vi "EPTxRTmul-inj2.0.vi"(0 "PatternConfig":T14 {"Max Rate [Hz]" format="%#_3p"}, 1 "EPTxFilters":T15={"Primary [s]"=5e-06, "Aux 1 [s]"=5e-06, "Aux 2 [s]"=0.0, "Aux 3 [s]"=0.0, "Aux 4 [s]"=0.0} {"Aux 4 [s]" format="%#_6p"; "Aux 3 [s]" format="%#_6p"; "Aux 2 [s]" format="%#_6p"; "Aux 1 [s]" format="%#_6p"; "Primary [s]" format="%#_6p"}, 5 "RT_Input":T4={"Load"=FALSE, "History_[CAD]"=63, "Stall_Speed_[RPM]"=200.0, "Delay_time[ms]"=0.0} caption="簇", 9 "EPTxState":T17={"Sync Enable"=TRUE, "Clear Errors"=FALSE, "Sim Enable"=FALSE, "Sim Speed [RPM]"=1000.0}, 11 "SimulatorConfig":T13={"Sim Speed [RPM]"=1000.0, "Ramp Rate [RPM/s]"=50.0, "Rotations"=2, "Pause"=FALSE, "Pause Angle [CAD]"=0.0, "Max Offset [RPM]"=0.0, "Cylinders"=6}, 12 "EPTxSupervisor_rt":T9={"Sync"=FALSE, "CurrentCAD"=0.0, "MaxCAD"=720.0, "HistoryCAD"=61.0, "CADRate"=0.0, "AvgSpeed"=0.0, "Config"=FALSE, "Rcvg Primary"=FALSE, "Stall"=FALSE, "Overflow"=FALSE, "Ratio Error"=FALSE, "Pattern Error"=FALSE, "Aux Warning"=FALSE, "Watchdog Error"=FALSE}, 13 "Control_strategy_input":T3={"Injection_DBTDC"=6.0, "Injection_duration[ms]"=2.0} caption="簇") -> (3 "EPTxControl":T10={"Sync Enable"=FALSE, "Clear Errors"=FALSE, "Sim Enable"=FALSE, "Sim Rate"=63.999996185302734, "Watchdog"=FALSE}, 4 "Config_number":T7 caption="簇", 6 "Lighting":T8 caption="簇", 10 "EPTxPatternConfig":T11 {"Pattern"."Aux 4" format="%#_16g"; "Pattern"."Aux 3" format="%#_16g"; "Pattern"."Aux 2" format="%#_16g"; "Pattern"."Aux 1" format="%#_16g"; "Pattern"."Primary" format="%#_16g"}, 14 "CylinderSig":T2={"CylinderSig_1"={"Cylinder1_H_R[CAD]"=204.0, "Cylinder1_H_F[CAD]"=210.0}, "CylinderSig_2"={"Cylinder2_H_R[CAD]"=684.0, "Cylinder2_H_F[CAD]"=690.0}, "CylinderSig_3"={"Cylinder3_H_R[CAD]"=444.0, "Cylinder3_H_F[CAD]"=450.0}, "CylinderSig_4"={"Cylinder4_H_R[CAD]"=90.0, "Cylinder4_H_F[CAD]"=100.0}, "CylinderSig_5"={"Cylinder5_H_R[CAD]"=324.0, "Cylinder5_H_F[CAD]"=330.0}, "CylinderSig_6"={"Cylinder6_H_R[CAD]"=0.0, "Cylinder6_H_F[CAD]"=0.0}} caption="簇", 15 "Tick_output":T1 caption="簇")   [LabVIEW 2022 SP3]
uses:
  <vilib>/Powertrain Controls/Device Drivers/Engine Position Tracking/EPTx/RevA/RT/Controls/EPTxState.ctl
  <vilib>/Powertrain Controls/Device Drivers/Engine Position Tracking/EPTx/RevA/RT/Controls/EPTxData.ctl
  <vilib>/Powertrain Controls/Device Drivers/Engine Position Tracking/EPTx/RevA/RT/Controls/EPTxFilters.ctl
  <vilib>/Powertrain Controls/Device Drivers/Engine Position Tracking/EPTx/RevA/RT/Controls/Pattern Config.ctl
  <vilib>/Powertrain Controls/Device Drivers/Engine Position Tracking/EPTx/RevA/RT/Controls/Simulator Config.ctl
  <vilib>/Powertrain Controls/Device Drivers/Engine Position Tracking/EPTx/RevA/FPGA/Controls/EPTxPatternConfig.ctl
  <vilib>/Powertrain Controls/Device Drivers/Engine Position Tracking/EPTx/RevA/FPGA/Controls/Patterns.ctl
  <vilib>/Powertrain Controls/Device Drivers/Engine Position Tracking/EPTx/RevA/FPGA/Controls/EPTxControl.ctl
  <vilib>/Powertrain Controls/Device Drivers/Engine Position Tracking/EPTx/RevA/FPGA/Controls/EPTxSupervisor.ctl
  <vilib>/Powertrain Controls/Device Drivers/Engine Position Tracking/EPTx/RevA/FPGA/Controls/EPTxConfig.ctl
  <vilib>/Powertrain Controls/Device Drivers/Engine Position Tracking/EPTx/RevA/FPGA/Controls/EPTxSimulatorConfig.ctl
  <vilib>/Powertrain Controls/Device Drivers/Engine Position Tracking/EPTx/RevA/RT/Controls/EPTxPattern.ctl
  <vilib>/Powertrain Controls/Device Drivers/Engine Position Tracking/EPTx/RevA/RT/Controls/Pattern.ctl
  <vilib>/Powertrain Controls/Device Drivers/Engine Position Tracking/EPTx/RevA/RT/Controls/EPTxSettings.ctl
  <vilib>/Powertrain Controls/Device Drivers/Engine Position Tracking/EPTx/RevA/RT/Controls/Settings - Tooth.ctl
  <vilib>/Powertrain Controls/Device Drivers/Engine Position Tracking/EPTx/RevA/RT/Controls/Direction Detection.ctl
  <vilib>/Powertrain Controls/Device Drivers/Engine Position Tracking/EPTx/RevA/RT/Controls/Settings - Pattern.ctl
  <vilib>/Powertrain Controls/Device Drivers/Engine Position Tracking/EPTx/RevA/RT/Controls/Settings - Token.ctl
  <vilib>/Powertrain Controls/Device Drivers/Engine Position Tracking/EPTx/RevA/RT/Controls/Aux Signal.ctl
  <vilib>/Powertrain Controls/Device Drivers/Engine Position Tracking/EPTx/RevA/RT/Controls/Aux Type.ctl
  <vilib>/Powertrain Controls/Device Drivers/Engine Position Tracking/EPTx/RevA/RT/Controls/Aux Threshold.ctl
  <vilib>/Powertrain Controls/Device Drivers/Engine Position Tracking/EPTx/RevA/RT/EPTx - RevA - RT.lvlib
  <vilib>/Powertrain Controls/Device Drivers/Engine Position Tracking/EPTx/RevA/FPGA/EPTx - RevA - FPGA.lvlib
panel:
  out "EPTxData":T16={"Sync"=TRUE, "CurrentCAD"=122.91406, "Speed [RPM]"=999.75, "Config"=FALSE, "Rcvg Primary"=TRUE, "Stall"=FALSE, "Overflow"=FALSE, "Ratio Error"=FALSE, "Pattern Error"=FALSE, "Aux Warning"=FALSE, "Watchdog Error"=FALSE}
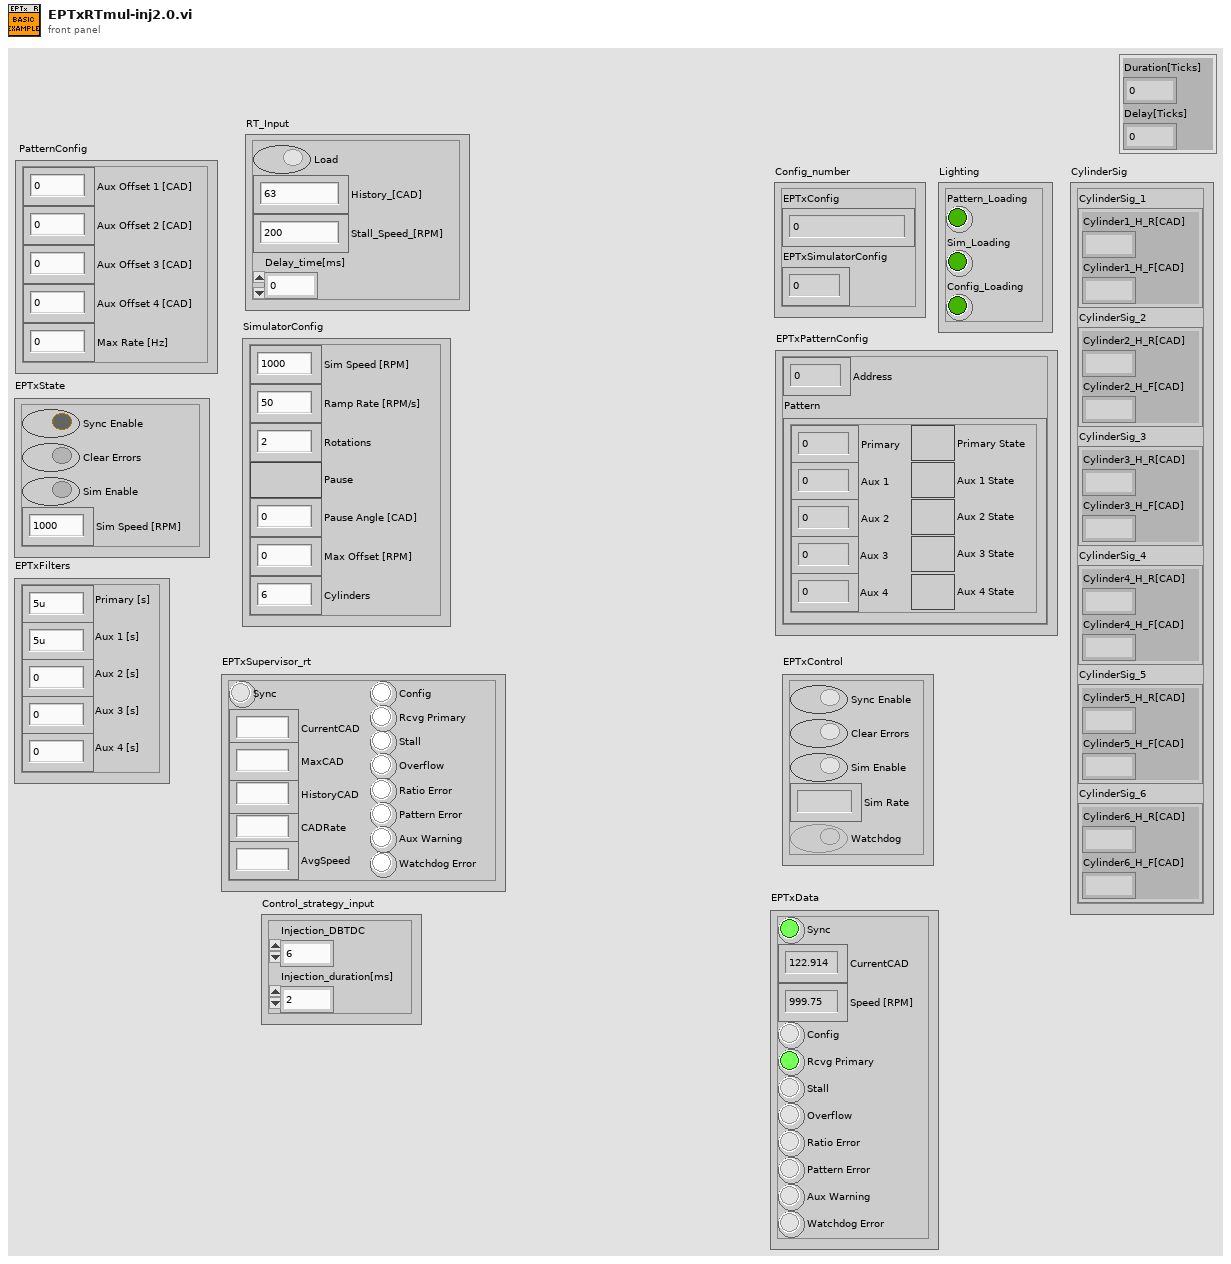
[diagram p1: front panel]
types:
  T1 = cluster{"Duration[Ticks]":u16, "Delay[Ticks]":u16}
  T2 = cluster{"CylinderSig_1":cluster{"Cylinder1_H_R[CAD]":fxp<+,18,11>, "Cylinder1_H_F[CAD]":fxp<+,18,11>}, "CylinderSig_2":cluster{"Cylinder2_H_R[CAD]":fxp<+,18,11>, "Cylinder2_H_F[CAD]":fxp<+,18,11>}, "CylinderSig_3":cluster{"Cylinder3_H_R[CAD]":fxp<+,18,11>, "Cylinder3_H_F[CAD]":fxp<+,18,11>}, "CylinderSig_4":cluster{"Cylinder4_H_R[CAD]":fxp<+,18,11>, "Cylinder4_H_F[CAD]":fxp<+,18,11>}, "CylinderSig_5":cluster{"Cylinder5_H_R[CAD]":fxp<+,18,11>, "Cylinder5_H_F[CAD]":fxp<+,18,11>}, "CylinderSig_6":cluster{"Cylinder6_H_R[CAD]":fxp<+,18,11>, "Cylinder6_H_F[CAD]":fxp<+,18,11>}}
  T3 = cluster{"Injection_DBTDC":sgl, "Injection_duration[ms]":sgl}
  T4 = cluster{"Load":bool, "History_[CAD]":u8, "Stall_Speed_[RPM]":sgl, "Delay_time[ms]":sgl}
  T5 = typedef "EPTx - RevA - FPGA.lvlib/EPTxConfig.ctl" = u64
  T6 = typedef "EPTx - RevA - FPGA.lvlib/EPTxSimulatorConfig.ctl" = u32
  T7 = cluster{"EPTxConfig":T5, "EPTxSimulatorConfig":T6}
  T8 = cluster{"Pattern_Loading":bool, "Sim_Loading":bool, "Config_Loading":bool}
  T9 = typedef "EPTx - RevA - FPGA.lvlib/EPTxSupervisor.ctl" = cluster{"Sync":bool, "CurrentCAD":fxp<+,18,11>, "MaxCAD":fxp<+,11,11>, "HistoryCAD":fxp<+,11,11>, "CADRate":fxp<+,22,8>, "AvgSpeed":fxp<+,17,15>, "Config":bool, "Rcvg Primary":bool, "Stall":bool, "Overflow":bool, "Ratio Error":bool, "Pattern Error":bool, "Aux Warning":bool, "Watchdog Error":bool}
  T10 = typedef "EPTx - RevA - FPGA.lvlib/EPTxControl.ctl" = cluster{"Sync Enable":bool, "Clear Errors":bool, "Sim Enable":bool, "Sim Rate":fxp<+,24,6>, "Watchdog":bool}
  T11 = typedef "EPTx - RevA - FPGA.lvlib/EPTxPatternConfig.ctl" = cluster{"Address":fxp<+,14,14>, "Pattern":T12}
  T12 = typedef "EPTx - RevA - FPGA.lvlib/Patterns.ctl" = cluster{"Primary":fxp<+,19,12>, "Primary State":bool, "Aux 1":fxp<+,19,12>, "Aux 1 State":bool, "Aux 2":fxp<+,19,12>, "Aux 2 State":bool, "Aux 3":fxp<+,19,12>, "Aux 3 State":bool, "Aux 4":fxp<+,19,12>, "Aux 4 State":bool}
  T13 = typedef "EPTx - RevA - RT.lvlib/Simulator Config.ctl" = cluster{"Sim Speed [RPM]":sgl, "Ramp Rate [RPM/s]":sgl, "Rotations":u8, "Pause":bool, "Pause Angle [CAD]":sgl, "Max Offset [RPM]":sgl, "Cylinders":u8}
  T14 = typedef "EPTx - RevA - RT.lvlib/Pattern Config.ctl" = cluster{"Aux Offset 1 [CAD]":sgl, "Aux Offset 2 [CAD]":sgl, "Aux Offset 3 [CAD]":sgl, "Aux Offset 4 [CAD]":sgl, "Max Rate [Hz]":sgl}
  T15 = typedef "EPTx - RevA - RT.lvlib/EPTxFilters.ctl" = cluster{"Primary [s]":sgl, "Aux 1 [s]":sgl, "Aux 2 [s]":sgl, "Aux 3 [s]":sgl, "Aux 4 [s]":sgl}
  T16 = typedef "EPTx - RevA - RT.lvlib/EPTxData.ctl" = cluster{"Sync":bool, "CurrentCAD":sgl, "Speed [RPM]":sgl, "Config":bool, "Rcvg Primary":bool, "Stall":bool, "Overflow":bool, "Ratio Error":bool, "Pattern Error":bool, "Aux Warning":bool, "Watchdog Error":bool}
  T17 = typedef "EPTx - RevA - RT.lvlib/EPTxState.ctl" = cluster{"Sync Enable":bool, "Clear Errors":bool, "Sim Enable":bool, "Sim Speed [RPM]":sgl}
  T18 = cluster{"CylinderSig_1":cluster{"Cylinder1_H_R [CAD]":fxp<+,18,11>, "Cylinder1_H_F [CAD]":fxp<+,18,11>}, "CylinderSig_2":cluster{"Cylinder2_H_R [CAD]":fxp<+,18,11>, "Cylinder2_H_F [CAD]":fxp<+,18,11>}, "CylinderSig_3":cluster{"Cylinder3_H_R [CAD]":fxp<+,18,11>, "Cylinder3_H_F [CAD]":fxp<+,18,11>}, "CylinderSig_4":cluster{"Cylinder4_H_R [CAD]":fxp<+,18,11>, "Cylinder4_H_F [CAD]":fxp<+,18,11>}, "CylinderSig_5":cluster{"Cylinder5_H_R [CAD]":fxp<+,18,11>, "Cylinder5_H_F [CAD]":fxp<+,18,11>}, "CylinderSig_6":cluster{"Cylinder6_H_R [CAD]":fxp<+,18,11>, "Cylinder6_H_F [CAD]":fxp<+,18,11>}}
  T19 = cluster{"Cylinder6_H_R [CAD]":fxp<+,18,11>, "Cylinder6_H_F [CAD]":fxp<+,18,11>}
  T20 = cluster{"Cylinder5_H_R [CAD]":fxp<+,18,11>, "Cylinder5_H_F [CAD]":fxp<+,18,11>}
  T21 = cluster{"Cylinder4_H_R [CAD]":fxp<+,18,11>, "Cylinder4_H_F [CAD]":fxp<+,18,11>}
  T22 = cluster{"Cylinder3_H_R [CAD]":fxp<+,18,11>, "Cylinder3_H_F [CAD]":fxp<+,18,11>}
  T23 = cluster{"Cylinder2_H_R [CAD]":fxp<+,18,11>, "Cylinder2_H_F [CAD]":fxp<+,18,11>}
  T24 = cluster{"Cylinder1_H_R [CAD]":fxp<+,18,11>, "Cylinder1_H_F [CAD]":fxp<+,18,11>}
  T25 = cluster{"Pattern Loading":bool, "Sim Loading":bool, "Config Loading":bool}
  T26 = typedef "EPTx - RevA - RT.lvlib/EPTxSettings.ctl" = cluster{"Rotation":u8, "Ratios":sgl[], "Thresholds":sgl[], "Tooth":T27, "Pattern":T29[], "Token":T30[], "Aux Threshold Min":T33, "Aux Threshold Max":T33}
  T27 = typedef "EPTx - RevA - RT.lvlib/Settings - Tooth.ctl" = cluster{"Rising Edge":bool, "Falling Edge":bool, "Direction\nDetection":T28, "Level":bool, "Parameter":sgl}
  T28 = typedef "EPTx - RevA - RT.lvlib/Direction Detection.ctl" = enum16{"None", "Aux Signal", "Length"}
  T29 = typedef "EPTx - RevA - RT.lvlib/Settings - Pattern.ctl" = cluster{"Ratio Index":u8, "Ratio Count":u16, "Angle":sgl, "dAngle":sgl}
  T30 = typedef "EPTx - RevA - RT.lvlib/Settings - Token.ctl" = cluster{"Length":u16, "Start Index":u8, "Start Count":u16, "Aux 1":T31, "Aux 1 Type":T32, "Aux 1 Max":u16, "Aux 1 Min":u16, "Aux 2":T31, "Aux 2 Type":T32, "Aux 2 Max":u16, "Aux 2 Min":u16, "End Index":u8, "End Count":u16}
  T31 = typedef "EPTx - RevA - RT.lvlib/Aux Signal.ctl" = enum8{"---", "Aux 1", "Aux 2", "Aux 3", "Aux 4"}
  T32 = typedef "EPTx - RevA - RT.lvlib/Aux Type.ctl" = enum8{"Falling", "Rising", "Low", "High", "Ratio"}
  T33 = typedef "EPTx - RevA - RT.lvlib/Aux Threshold.ctl" = cluster{"Aux 1":sgl, "Aux 2":sgl, "Aux 3":sgl, "Aux 4":sgl}
  T34 = typedef "EPTx - RevA - RT.lvlib/EPTxPattern.ctl" = cluster{"Rotations":u8, "Cylinders":u8, "Primary":T35[], "Aux 1":T35[], "Aux 2":T35[], "Aux 3":T35[], "Aux 4":T35[]}
  T35 = typedef "EPTx - RevA - RT.lvlib/Pattern.ctl" = cluster{"Angle":sgl, "State":bool}
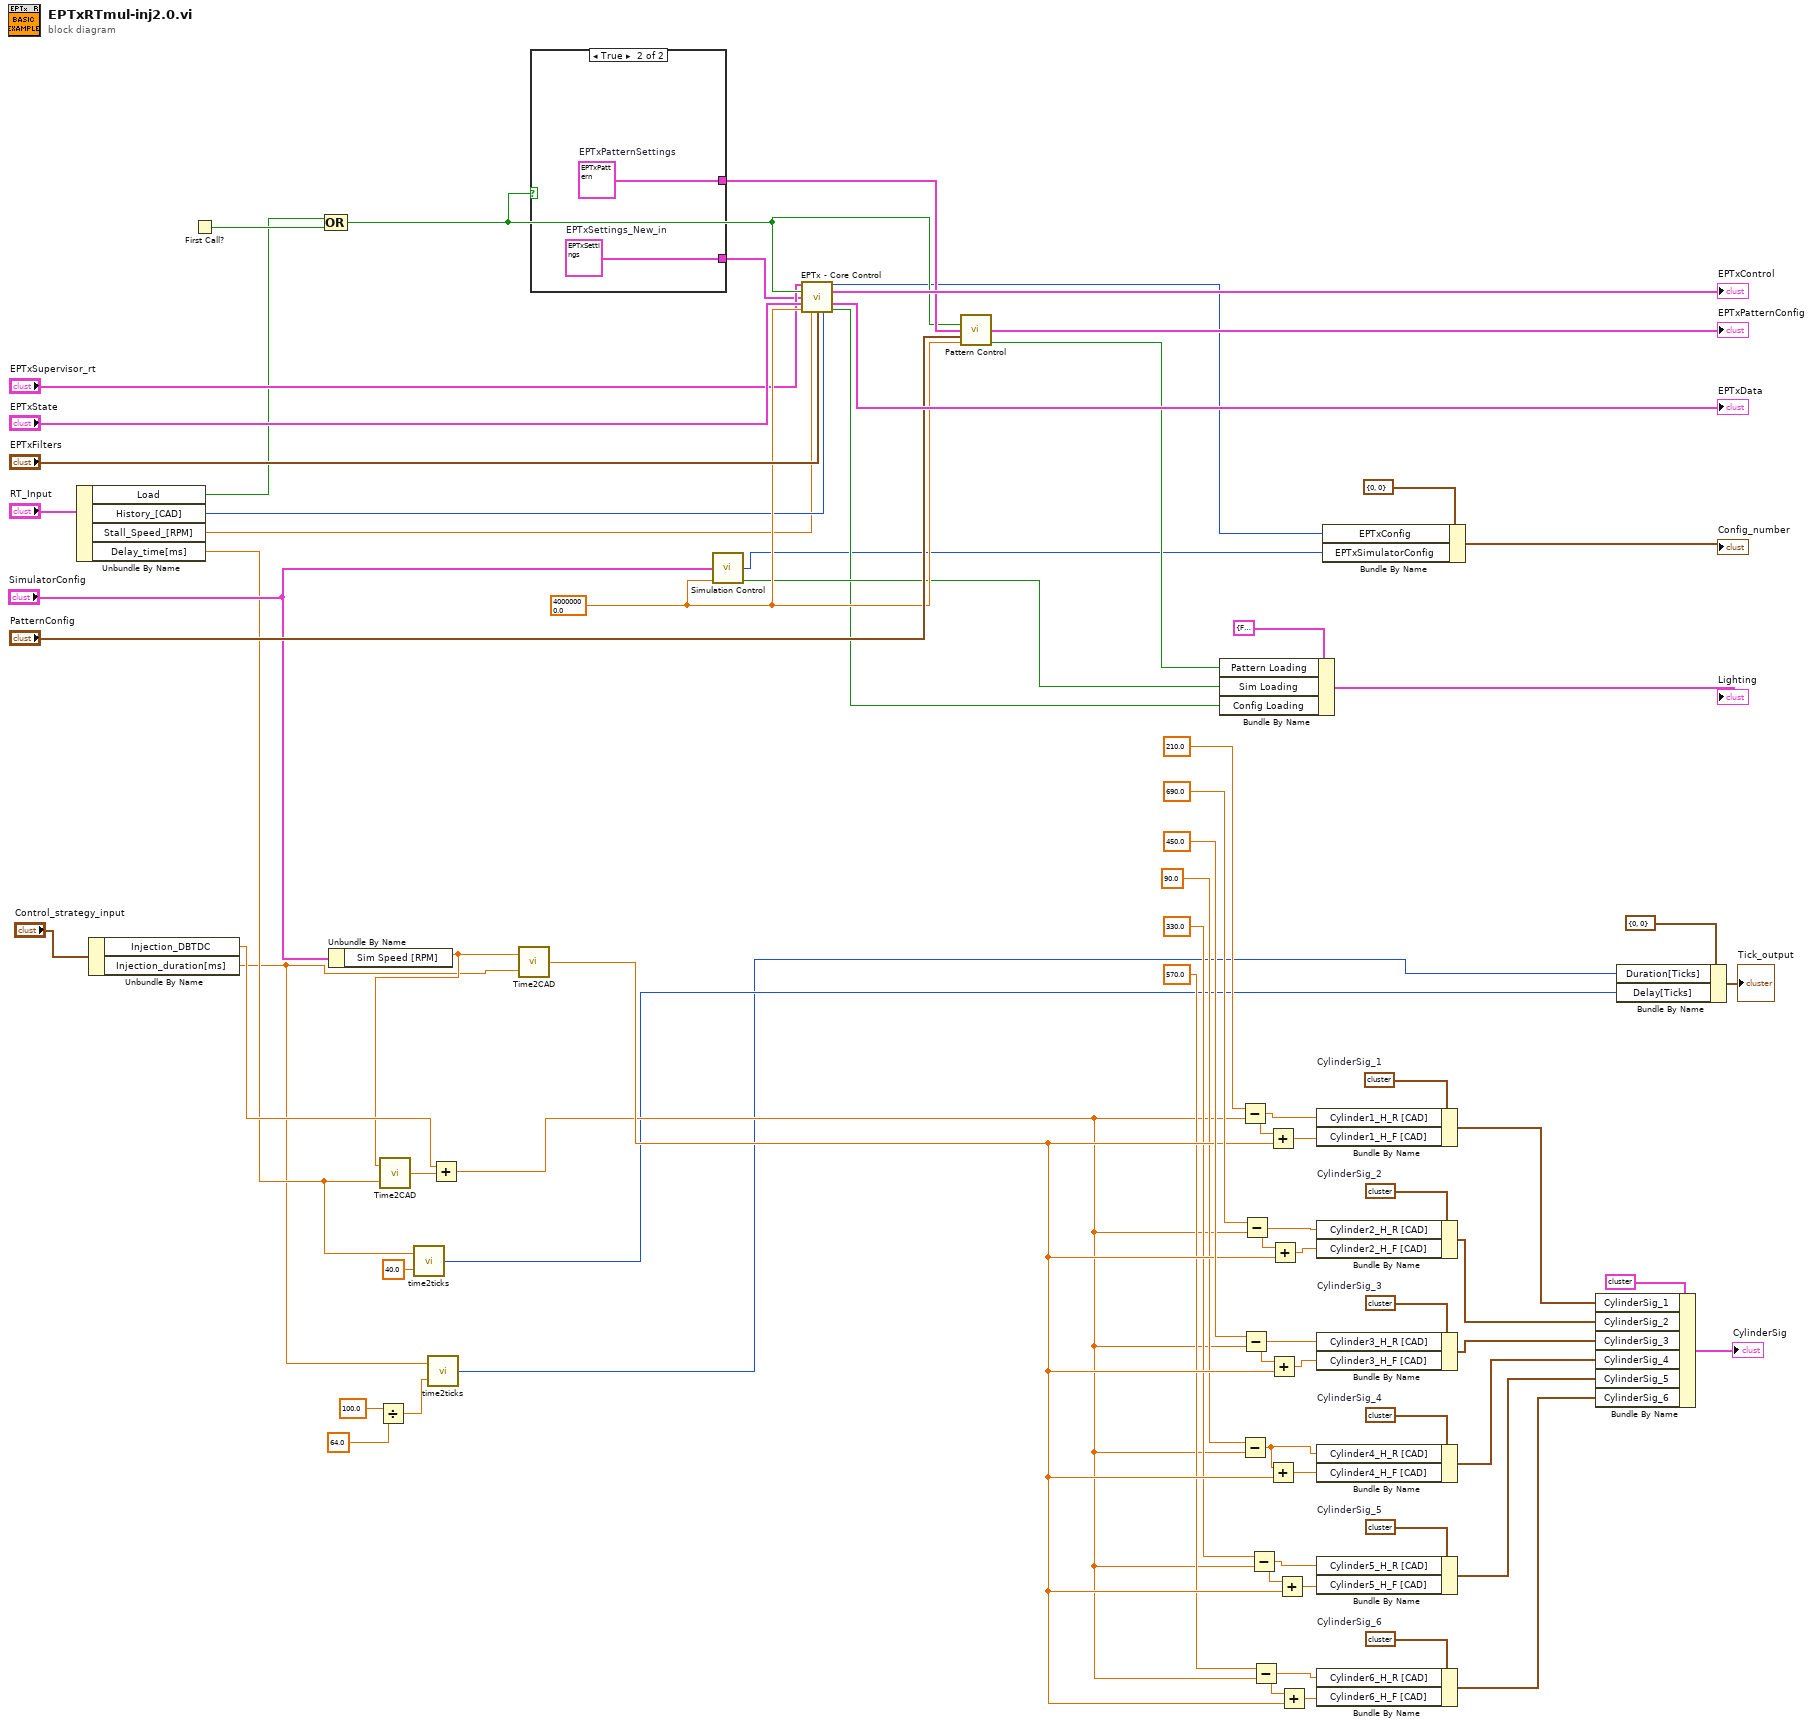
[diagram p0: block diagram]
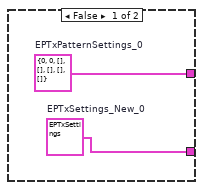
[diagram p2: hidden frame]
diagram:
  w43 = T19 {"Cylinder6_H_R [CAD]"=0.0, "Cylinder6_H_F [CAD]"=0.0}  # CylinderSig_6
  w44 = T20 {"Cylinder5_H_R [CAD]"=324.0, "Cylinder5_H_F [CAD]"=330.0}  # CylinderSig_5
  w45 = T21 {"Cylinder4_H_R [CAD]"=90.0, "Cylinder4_H_F [CAD]"=100.0}  # CylinderSig_4
  w46 = T22 {"Cylinder3_H_R [CAD]"=444.0, "Cylinder3_H_F [CAD]"=450.0}  # CylinderSig_3
  w47 = T23 {"Cylinder2_H_R [CAD]"=684.0, "Cylinder2_H_F [CAD]"=690.0}  # CylinderSig_2
  w48 = T24 {"Cylinder1_H_R [CAD]"=204.0, "Cylinder1_H_F [CAD]"=210.0}  # CylinderSig_1
  w68 = sgl 40000000.0 ("Frequency (40M) [Hz]")
  n1 = Unbundle By Name("RT_Input") -> ("Load"=w53:bool, "History_[CAD]"=w52:u8, "Stall_Speed_[RPM]"=w51:sgl, "Delay_time[ms]"=w10:sgl)
  n2 = Unbundle By Name("Control_strategy_input") -> ("Injection_DBTDC"=w14:sgl, "Injection_duration[ms]"=w9:sgl)
  n3 = First Call?() -> (First Call?: T/F=w66:bool)
  n4 = Compound Arithmetic op=OR ("复合运算")(w53, w66) -> (w65:bool)
  n5 = Unbundle By Name("SimulatorConfig") -> ("Sim Speed [RPM]"=w12:sgl)
  n6 = Divide(x=100.0, y=64.0) -> (x/y=w1:dbl)
  n7 = call <vilib>:"Time2CAD.vi"("Time [ms]"=w10, "Speed (RPM)"=w12) -> ("CAD"=w11:sgl)
  n8 = call <vilib>:"time2ticks.vi"("Clock Frequency (MHz, 40)"=sgl 40.0, "Time (msec)"=w10) -> ("Ticks"=w6:u32)
  n9 = call <vilib>:"time2ticks.vi"("Clock Frequency (MHz, 40)"=w1, "Time (msec)"=w9) -> ("Ticks"=w5:u32)
  n10 = Add(x=w14, y=w11) -> (x+y=w13:sgl)
  n11 = call <vilib>:"Time2CAD.vi"("Time [ms]"=w9, "Speed (RPM)"=w12) -> ("CAD"=w30:sgl)
  n12 = case shown="True" w65 {
    tunnel: [w76 w78] -> w67
    tunnel: [w75 w77] -> w15
    frame False {
      w75 = T26 {"Rotation"=0, "Ratios"=[], "Thresholds"=[], "Tooth"={"Rising Edge"=FALSE, "Falling Edge"=FALSE, "Direction\nDetection"=enum."None", "Level"=FALSE, "Parameter"=0.0}, "Pattern"=[], "Token"=[], "Aux Threshold Min"={"Aux 1"=0.0, "Aux 2"=0.0, "Aux 3"=0.0, "Aux 4"=0.0}, "Aux Threshold Max"={"Aux 1"=0.0, "Aux 2"=0.0, "Aux 3"=0.0, "Aux 4"=0.0}}  # EPTxSettings_New_0
      w76 = T34 {"Rotations"=0, "Cylinders"=0, "Primary"=[], "Aux 1"=[], "Aux 2"=[], "Aux 3"=[], "Aux 4"=[]}  # EPTxPatternSettings_0
    }
    frame True {
      w77 = T26 {"Rotation"=2, "Ratios"=[0.33333334, 1.0, 3.0], "Thresholds"=[0.16666667, 0.6666667, 0.6666667, 2.0, 2.0, 4.0, 999.0], "Tooth"={"Rising Edge"=TRUE, "Falling Edge"=FALSE, "Direction\nDetection"=enum."None", "Level"=FALSE, "Parameter"=0.0}, "Pattern"=[{"Ratio Index"=0, "Ratio Count"=1, "Angle"=0.0, "dAngle"=6.0}, {"Ratio Index"=1, "Ratio Count"=56, "Angle"=6.0, "dAngle"=6.0}, {"Ratio Index"=2, "Ratio Count"=1, "Angle"=342.0, "dAngle"=18.0}, {"Ratio Index"=0, "Ratio Count"=1, "Angle"=360.0, "dAngle"=6.0}, {"Ratio Index"=1, "Ratio Count"=56, "Angle"=366.0, "dAngle"=6.0}, {"Ratio Index"=2, "Ratio Count"=1, "Angle"=702.0, "dAngle"=18.0}], "Token"=[{"Length"=1, "Start Index"=5, "Start Count"=0, "Aux 1"=enum."---", "Aux 1 Type"=enum."Falling", "Aux 1 Max"=0, "Aux 1 Min"=0, "Aux 2"=enum."Aux 2", "Aux 2 Type"=enum."Ratio", "Aux 2 Max"=73, "Aux 2 Min"=73, "End Index"=0, "End Count"=0}], "Aux Threshold Min"={"Aux 1"=1.8809524, "Aux 2"=1.2142857, "Aux 3"=0.0, "Aux 4"=0.0}, "Aux Threshold Max"={"Aux 1"=2.7857144, "Aux 2"=1.8809524, "Aux 3"=999.0, "Aux 4"=999.0}}  # EPTxSettings_New_in
      w78 = T34 {"Rotations"=2, "Cylinders"=6, "Primary"=[{"Angle"=0.0, "State"=FALSE}, {"Angle"=3.0, "State"=TRUE}, {"Angle"=6.0, "State"=FALSE}, {"Angle"=9.0, "State"=TRUE}, {"Angle"=12.0, "State"=FALSE}, {"Angle"=15.0, "State"=TRUE}, {"Angle"=18.0, "State"=FALSE}, {"Angle"=21.0, "State"=TRUE}, {"Angle"=24.0, "State"=FALSE}, {"Angle"=27.0, "State"=TRUE}, {"Angle"=30.0, "State"=FALSE}, {"Angle"=33.0, "State"=TRUE}, {"Angle"=36.0, "State"=FALSE}, {"Angle"=39.0, "State"=TRUE}, {"Angle"=42.0, "State"=FALSE}, {"Angle"=45.0, "State"=TRUE}, {"Angle"=48.0, "State"=FALSE}, {"Angle"=51.0, "State"=TRUE}, {"Angle"=54.0, "State"=FALSE}, {"Angle"=57.0, "State"=TRUE}, {"Angle"=60.0, "State"=FALSE}, {"Angle"=63.0, "State"=TRUE}, {"Angle"=66.0, "State"=FALSE}, {"Angle"=69.0, "State"=TRUE}, {"Angle"=72.0, "State"=FALSE}, {"Angle"=75.0, "State"=TRUE}, {"Angle"=78.0, "State"=FALSE}, {"Angle"=81.0, "State"=TRUE}, {"Angle"=84.0, "State"=FALSE}, {"Angle"=87.0, "State"=TRUE}, {"Angle"=90.0, "State"=FALSE}, {"Angle"=93.0, "State"=TRUE}, {"Angle"=96.0, "State"=FALSE}, {"Angle"=99.0, "State"=TRUE}, {"Angle"=102.0, "State"=FALSE}, {"Angle"=105.0, "State"=TRUE}, {"Angle"=108.0, "State"=FALSE}, {"Angle"=111.0, "State"=TRUE}, {"Angle"=114.0, "State"=FALSE}, {"Angle"=117.0, "State"=TRUE}, {"Angle"=120.0, "State"=FALSE}, {"Angle"=123.0, "State"=TRUE}, {"Angle"=126.0, "State"=FALSE}, {"Angle"=129.0, "State"=TRUE}, {"Angle"=132.0, "State"=FALSE}, {"Angle"=135.0, "State"=TRUE}, {"Angle"=138.0, "State"=FALSE}, {"Angle"=141.0, "State"=TRUE}, {"Angle"=144.0, "State"=FALSE}, {"Angle"=147.0, "State"=TRUE}, {"Angle"=150.0, "State"=FALSE}, {"Angle"=153.0, "State"=TRUE}, {"Angle"=156.0, "State"=FALSE}, {"Angle"=159.0, "State"=TRUE}, {"Angle"=162.0, "State"=FALSE}, {"Angle"=165.0, "State"=TRUE}, {"Angle"=168.0, "State"=FALSE}, {"Angle"=171.0, "State"=TRUE}, {"Angle"=174.0, "State"=FALSE}, {"Angle"=177.0, "State"=TRUE}, {"Angle"=180.0, "State"=FALSE}, {"Angle"=183.0, "State"=TRUE}, {"Angle"=186.0, "State"=FALSE}, {"Angle"=189.0, "State"=TRUE}, {"Angle"=192.0, "State"=FALSE}, {"Angle"=195.0, "State"=TRUE}, {"Angle"=198.0, "State"=FALSE}, {"Angle"=201.0, "State"=TRUE}, {"Angle"=204.0, "State"=FALSE}, {"Angle"=207.0, "State"=TRUE}, {"Angle"=210.0, "State"=FALSE}, {"Angle"=213.0, "State"=TRUE}, {"Angle"=216.0, "State"=FALSE}, {"Angle"=219.0, "State"=TRUE}, {"Angle"=222.0, "State"=FALSE}, {"Angle"=225.0, "State"=TRUE}, {"Angle"=228.0, "State"=FALSE}, {"Angle"=231.0, "State"=TRUE}, {"Angle"=234.0, "State"=FALSE}, {"Angle"=237.0, "State"=TRUE}, {"Angle"=240.0, "State"=FALSE}, {"Angle"=243.0, "State"=TRUE}, {"Angle"=246.0, "State"=FALSE}, {"Angle"=249.0, "State"=TRUE}, {"Angle"=252.0, "State"=FALSE}, {"Angle"=255.0, "State"=TRUE}, {"Angle"=258.0, "State"=FALSE}, {"Angle"=261.0, "State"=TRUE}, {"Angle"=264.0, "State"=FALSE}, {"Angle"=267.0, "State"=TRUE}, {"Angle"=270.0, "State"=FALSE}, {"Angle"=273.0, "State"=TRUE}, {"Angle"=276.0, "State"=FALSE}, {"Angle"=279.0, "State"=TRUE}, {"Angle"=282.0, "State"=FALSE}, {"Angle"=285.0, "State"=TRUE}, {"Angle"=288.0, "State"=FALSE}, {"Angle"=291.0, "State"=TRUE}, {"Angle"=294.0, "State"=FALSE}, {"Angle"=297.0, "State"=TRUE}, {"Angle"=300.0, "State"=FALSE}, {"Angle"=303.0, "State"=TRUE}, {"Angle"=306.0, "State"=FALSE}, {"Angle"=309.0, "State"=TRUE}, {"Angle"=312.0, "State"=FALSE}, {"Angle"=315.0, "State"=TRUE}, {"Angle"=318.0, "State"=FALSE}, {"Angle"=321.0, "State"=TRUE}, {"Angle"=324.0, "State"=FALSE}, {"Angle"=327.0, "State"=TRUE}, {"Angle"=330.0, "State"=FALSE}, {"Angle"=333.0, "State"=TRUE}, {"Angle"=336.0, "State"=FALSE}, {"Angle"=339.0, "State"=TRUE}, {"Angle"=342.0, "State"=FALSE}, {"Angle"=345.0, "State"=TRUE}, {"Angle"=360.0, "State"=FALSE}, {"Angle"=363.0, "State"=TRUE}, {"Angle"=366.0, "State"=FALSE}, {"Angle"=369.0, "State"=TRUE}, {"Angle"=372.0, "State"=FALSE}, {"Angle"=375.0, "State"=TRUE}, {"Angle"=378.0, "State"=FALSE}, {"Angle"=381.0, "State"=TRUE}, {"Angle"=384.0, "State"=FALSE}, {"Angle"=387.0, "State"=TRUE}, {"Angle"=390.0, "State"=FALSE}, {"Angle"=393.0, "State"=TRUE}, {"Angle"=396.0, "State"=FALSE}, {"Angle"=399.0, "State"=TRUE}, {"Angle"=402.0, "State"=FALSE}, {"Angle"=405.0, "State"=TRUE}, {"Angle"=408.0, "State"=FALSE}, {"Angle"=411.0, "State"=TRUE}, {"Angle"=414.0, "State"=FALSE}, {"Angle"=417.0, "State"=TRUE}, {"Angle"=420.0, "State"=FALSE}, {"Angle"=423.0, "State"=TRUE}, {"Angle"=426.0, "State"=FALSE}, {"Angle"=429.0, "State"=TRUE}, {"Angle"=432.0, "State"=FALSE}, {"Angle"=435.0, "State"=TRUE}, {"Angle"=438.0, "State"=FALSE}, {"Angle"=441.0, "State"=TRUE}, {"Angle"=444.0, "State"=FALSE}, {"Angle"=447.0, "State"=TRUE}, {"Angle"=450.0, "State"=FALSE}, {"Angle"=453.0, "State"=TRUE}, {"Angle"=456.0, "State"=FALSE}, {"Angle"=459.0, "State"=TRUE}, {"Angle"=462.0, "State"=FALSE}, {"Angle"=465.0, "State"=TRUE}, {"Angle"=468.0, "State"=FALSE}, {"Angle"=471.0, "State"=TRUE}, {"Angle"=474.0, "State"=FALSE}, {"Angle"=477.0, "State"=TRUE}, {"Angle"=480.0, "State"=FALSE}, {"Angle"=483.0, "State"=TRUE}, {"Angle"=486.0, "State"=FALSE}, {"Angle"=489.0, "State"=TRUE}, {"Angle"=492.0, "State"=FALSE}, {"Angle"=495.0, "State"=TRUE}, {"Angle"=498.0, "State"=FALSE}, {"Angle"=501.0, "State"=TRUE}, {"Angle"=504.0, "State"=FALSE}, {"Angle"=507.0, "State"=TRUE}, {"Angle"=510.0, "State"=FALSE}, {"Angle"=513.0, "State"=TRUE}, {"Angle"=516.0, "State"=FALSE}, {"Angle"=519.0, "State"=TRUE}, {"Angle"=522.0, "State"=FALSE}, {"Angle"=525.0, "State"=TRUE}, {"Angle"=528.0, "State"=FALSE}, {"Angle"=531.0, "State"=TRUE}, {"Angle"=534.0, "State"=FALSE}, {"Angle"=537.0, "State"=TRUE}, {"Angle"=540.0, "State"=FALSE}, {"Angle"=543.0, "State"=TRUE}, {"Angle"=546.0, "State"=FALSE}, {"Angle"=549.0, "State"=TRUE}, {"Angle"=552.0, "State"=FALSE}, {"Angle"=555.0, "State"=TRUE}, {"Angle"=558.0, "State"=FALSE}, {"Angle"=561.0, "State"=TRUE}, {"Angle"=564.0, "State"=FALSE}, {"Angle"=567.0, "State"=TRUE}, {"Angle"=570.0, "State"=FALSE}, {"Angle"=573.0, "State"=TRUE}, {"Angle"=576.0, "State"=FALSE}, {"Angle"=579.0, "State"=TRUE}, {"Angle"=582.0, "State"=FALSE}, {"Angle"=585.0, "State"=TRUE}, {"Angle"=588.0, "State"=FALSE}, {"Angle"=591.0, "State"=TRUE}, {"Angle"=594.0, "State"=FALSE}, {"Angle"=597.0, "State"=TRUE}, {"Angle"=600.0, "State"=FALSE}, {"Angle"=603.0, "State"=TRUE}, {"Angle"=606.0, "State"=FALSE}, {"Angle"=609.0, "State"=TRUE}, {"Angle"=612.0, "State"=FALSE}, {"Angle"=615.0, "State"=TRUE}, {"Angle"=618.0, "State"=FALSE}, {"Angle"=621.0, "State"=TRUE}, {"Angle"=624.0, "State"=FALSE}, {"Angle"=627.0, "State"=TRUE}, {"Angle"=630.0, "State"=FALSE}, {"Angle"=633.0, "State"=TRUE}, {"Angle"=636.0, "State"=FALSE}, {"Angle"=639.0, "State"=TRUE}, {"Angle"=642.0, "State"=FALSE}, {"Angle"=645.0, "State"=TRUE}, {"Angle"=648.0, "State"=FALSE}, {"Angle"=651.0, "State"=TRUE}, {"Angle"=654.0, "State"=FALSE}, {"Angle"=657.0, "State"=TRUE}, {"Angle"=660.0, "State"=FALSE}, {"Angle"=663.0, "State"=TRUE}, {"Angle"=666.0, "State"=FALSE}, {"Angle"=669.0, "State"=TRUE}, {"Angle"=672.0, "State"=FALSE}, {"Angle"=675.0, "State"=TRUE}, {"Angle"=678.0, "State"=FALSE}, {"Angle"=681.0, "State"=TRUE}, {"Angle"=684.0, "State"=FALSE}, {"Angle"=687.0, "State"=TRUE}, {"Angle"=690.0, "State"=FALSE}, {"Angle"=693.0, "State"=TRUE}, {"Angle"=696.0, "State"=FALSE}, {"Angle"=699.0, "State"=TRUE}, {"Angle"=702.0, "State"=FALSE}, {"Angle"=705.0, "State"=TRUE}], "Aux 1"=[{"Angle"=12.0, "State"=TRUE}, {"Angle"=24.0, "State"=FALSE}, {"Angle"=48.0, "State"=TRUE}, {"Angle"=60.0, "State"=FALSE}, {"Angle"=132.0, "State"=TRUE}, {"Angle"=144.0, "State"=FALSE}, {"Angle"=198.0, "State"=TRUE}, {"Angle"=252.0, "State"=TRUE}, {"Angle"=264.0, "State"=FALSE}, {"Angle"=318.0, "State"=TRUE}, {"Angle"=372.0, "State"=TRUE}, {"Angle"=384.0, "State"=FALSE}, {"Angle"=438.0, "State"=TRUE}, {"Angle"=492.0, "State"=TRUE}, {"Angle"=504.0, "State"=FALSE}, {"Angle"=558.0, "State"=TRUE}, {"Angle"=612.0, "State"=TRUE}, {"Angle"=624.0, "State"=FALSE}, {"Angle"=678.0, "State"=TRUE}], "Aux 2"=[{"Angle"=12.0, "State"=TRUE}, {"Angle"=24.0, "State"=FALSE}, {"Angle"=48.0, "State"=TRUE}, {"Angle"=60.0, "State"=FALSE}, {"Angle"=132.0, "State"=TRUE}, {"Angle"=144.0, "State"=FALSE}, {"Angle"=198.0, "State"=TRUE}, {"Angle"=252.0, "State"=TRUE}, {"Angle"=264.0, "State"=FALSE}, {"Angle"=318.0, "State"=TRUE}, {"Angle"=372.0, "State"=TRUE}, {"Angle"=384.0, "State"=FALSE}, {"Angle"=438.0, "State"=TRUE}, {"Angle"=492.0, "State"=TRUE}, {"Angle"=504.0, "State"=FALSE}, {"Angle"=558.0, "State"=TRUE}, {"Angle"=612.0, "State"=TRUE}, {"Angle"=624.0, "State"=FALSE}, {"Angle"=678.0, "State"=TRUE}], "Aux 3"=[], "Aux 4"=[]}  # EPTxPatternSettings
    }
  }
  n13 = call <vilib>:"Simulation Control.vi"("SimulatorConfig"="SimulatorConfig", "Frequency (40M) [Hz]"=w68) -> ("EPTxSimulatorConfig"=w55:T6, "Loading"=w60:bool)  [unwired: 12 in]
  n14 = call <vilib>:"EPTx - Core Control.vi"("EPTxSupervisor"="EPTxSupervisor_rt", "Load"=w65, "EPTxSettings"=w15, "EPTxState"="EPTxState", "Frequency (40M) [Hz]"=w68, "Stall Speed (200) [RPM]"=w51, "Filters (0)"="EPTxFilters", "History (63) [CAD]"=w52) -> ("EPTxConfig"=w56:T5, "EPTxControl"=→"EPTxControl":T10, "EPTxData"=→"EPTxData":T16, "Loading"=w59:bool)  [unwired: 3 in, 1 out]
  n15 = call <vilib>:"Pattern Control.vi"("Load"=w65, "EPTxPatternSettings"=w67, "PatternConfig"="PatternConfig", "Frequency (40M) [Hz]"=w68) -> ("EPTxPatternConfig"=→"EPTxPatternConfig":T11, "Loading"=w62:bool)  [unwired: 10 in]
  n16 = Bundle By Name(cluster=T25 {"Pattern Loading"=FALSE, "Sim Loading"=FALSE, "Config Loading"=FALSE} ("Cluster"), "Pattern Loading"=w62, "Sim Loading"=w60, "Config Loading"=w59) -> (→"Lighting":T25)
  n17 = Subtract(x=sgl 210.0 ("Cylinder TDC [Absolute CAD]"), y=w13) -> (x-y=w40:sgl)
  n18 = Subtract(x=sgl 90.0 ("Cylinder TDC [Absolute CAD]"), y=w13) -> (x-y=w16:sgl)
  n19 = Subtract(x=sgl 450.0 ("Cylinder TDC [Absolute CAD]"), y=w13) -> (x-y=w35:sgl)
  n20 = Subtract(x=sgl 690.0 ("Cylinder TDC [Absolute CAD]"), y=w13) -> (x-y=w38:sgl)
  n21 = Subtract(x=sgl 330.0 ("Cylinder TDC [Absolute CAD]"), y=w13) -> (x-y=w17:sgl)
  n22 = Subtract(x=sgl 570.0 ("Cylinder TDC [Absolute CAD]"), y=w13) -> (x-y=w18:sgl)
  n23 = Add(x=w40, y=w30) -> (x+y=w41:sgl)
  n24 = Add(x=w16, y=w30) -> (x+y=w33:sgl)
  n25 = Add(x=w35, y=w30) -> (x+y=w36:sgl)
  n26 = Add(x=w38, y=w30) -> (x+y=w39:sgl)
  n27 = Add(x=w17, y=w30) -> (x+y=w32:sgl)
  n28 = Add(x=w18, y=w30) -> (x+y=w31:sgl)
  n29 = Bundle By Name(cluster=w48, "Cylinder1_H_R [CAD]"=w40, "Cylinder1_H_F [CAD]"=w41) -> (w24:T24)
  n30 = Bundle By Name(cluster=w47, "Cylinder2_H_R [CAD]"=w38, "Cylinder2_H_F [CAD]"=w39) -> (w23:T23)
  n31 = Bundle By Name(cluster=w46, "Cylinder3_H_R [CAD]"=w35, "Cylinder3_H_F [CAD]"=w36) -> (w22:T22)
  n32 = Bundle By Name(cluster=w45, "Cylinder4_H_R [CAD]"=w16, "Cylinder4_H_F [CAD]"=w33) -> (w21:T21)
  n33 = Bundle By Name(cluster=w44, "Cylinder5_H_R [CAD]"=w17, "Cylinder5_H_F [CAD]"=w32) -> (w20:T20)
  n34 = Bundle By Name(cluster=w43, "Cylinder6_H_R [CAD]"=w18, "Cylinder6_H_F [CAD]"=w31) -> (w19:T19)
  n35 = Bundle By Name(cluster=T7 {"EPTxConfig"=0, "EPTxSimulatorConfig"=0} ("Config_number"), "EPTxConfig"=w56, "EPTxSimulatorConfig"=w55) -> (→"Config_number":T7)
  n36 = Bundle By Name(cluster=T18 {"CylinderSig_1"={"Cylinder1_H_R [CAD]"=204.0, "Cylinder1_H_F [CAD]"=210.0}, "CylinderSig_2"={"Cylinder2_H_R [CAD]"=684.0, "Cylinder2_H_F [CAD]"=690.0}, "CylinderSig_3"={"Cylinder3_H_R [CAD]"=444.0, "Cylinder3_H_F [CAD]"=450.0}, "CylinderSig_4"={"Cylinder4_H_R [CAD]"=90.0, "Cylinder4_H_F [CAD]"=100.0}, "CylinderSig_5"={"Cylinder5_H_R [CAD]"=324.0, "Cylinder5_H_F [CAD]"=330.0}, "CylinderSig_6"={"Cylinder6_H_R [CAD]"=0.0, "Cylinder6_H_F [CAD]"=0.0}} ("CylinderSig"), "CylinderSig_1"=w24, "CylinderSig_2"=w23, "CylinderSig_3"=w22, "CylinderSig_4"=w21, "CylinderSig_5"=w20, "CylinderSig_6"=w19) -> (→"CylinderSig":T18)
  n37 = Bundle By Name(cluster=T1 {"Duration[Ticks]"=0, "Delay[Ticks]"=0} ("Tick_output"), "Duration[Ticks]"=w5, "Delay[Ticks]"=w6) -> (→"Tick_output":T1)
